vi "Run VI in SubPanel.vi"(8 "error in (no error)":errorcluster, 11 "SubPanel in":refnum<class "SubPanel.lvclass">) -> (0 "error out":errorcluster, 3 "SubPanel out":refnum<class "SubPanel.lvclass">)   [LabVIEW 2012, in "SubPanel.lvlib" / "SubPanel.lvclass"]
uses:
  SubPanel.lvclass
  SubPanel.lvclass/SubPanel.ctl
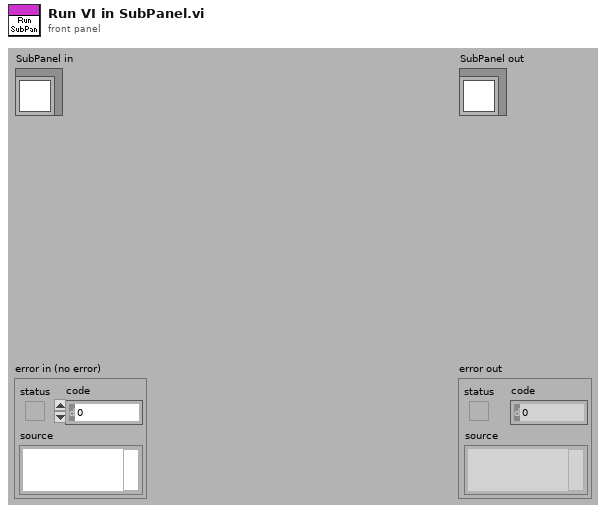
[diagram p1: front panel]
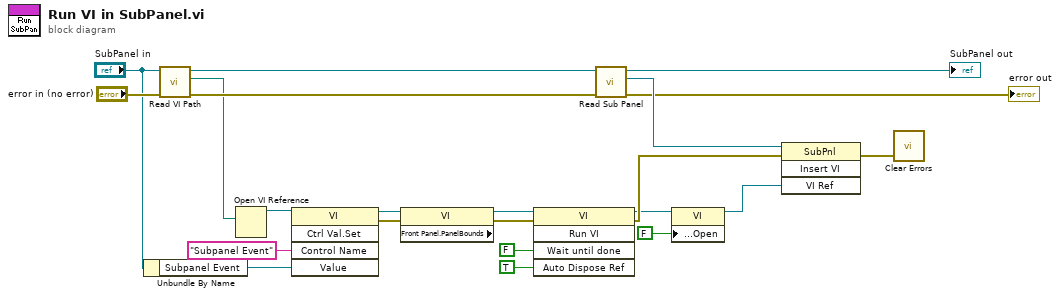
[diagram p0: block diagram]
diagram:
  n1 = Unbundle By Name("SubPanel in") -> ("Subpanel Event"=w2:refnum<user-event>)
  n2 = call-dynamic "Read VI Path.vi"("error in (no error)"="error in (no error)", "SubPanel.lvclass in"="SubPanel in") -> ("error out"=w21:errorcluster, "VI Path"=w4:path, "SubPanel.lvclass out"=w1:refnum<class "SubPanel.lvclass">)  [unwired: 7 out]
  n3 = Open VI Reference(vi path=w4) -> (vi reference=w17:refnum<vi>)  [unwired: 1 in, 5 out]
  n4 = invoke class="VI" method="Ctrl Val.Set"(reference=w17, "Control Name"="Subpanel Event", "Value"=w2) -> (reference out=w8:refnum<vi>, error out=w7:errorcluster)  [unwired: 2 in, 3 out]
  n5 = property class="VI" props=["Front Panel.PanelBounds"](reference=w8, error in=w7) -> (reference out=w6:refnum<vi>, error out=w5:errorcluster)  [unwired: 1 out]
  n6 = invoke class="VI" method="Run VI"(reference=w6, error in=w5, "Wait until done"=FALSE ("Wait Until Done"), "Auto Dispose Ref"=TRUE ("Auto Dispose Reference")) -> (reference out=w10:refnum<vi>, error out=w12:errorcluster)  [unwired: 1 in, 3 out]
  n7 = call-dynamic "Read Sub Panel.vi"("error in (no error)"=w21, "SubPanel.lvclass in"=w1) -> ("error out"=→"error out":errorcluster, "Sub Panel"=w19:refnum<vi>, "SubPanel.lvclass out"=→"SubPanel out":refnum<class "SubPanel.lvclass">)  [unwired: 7 out]
  n8 = property class="VI"(reference=w10, "Front Panel.Open"=FALSE ("Front Panel Window:Open")) -> (reference out=w9:refnum<vi>)  [unwired: 1 in, 1 out]
  n9 = invoke class="SubPnl" method="Insert VI"(reference=w19, error in=w12, "VI Ref"=w9) -> (error out=w18:errorcluster)  [unwired: 1 in, 3 out]
  n10 = call <vilib>:"Clear Errors.vi"("error in (no error)"=w18) -> ()  [unwired: 7 out]
